vi "Init SPI.vi"(6 "SPI Config":T1={"Mode"=0, "Data Bits"=8, "TX GPIO"=7, "RX GPIO"=4, "SCK GPIO"=6}, 7 "SPI #":T4=-1, 8 "error in (no error)":errorcluster, 10 "Baud":u32=1000000 format="%.0p", 11 "VisaSession in":refnum<class "VisaSession.lvclass">) -> (0 "error out":errorcluster, 2 "SPI":refnum<class "SPI.lvclass">, 3 "VisaSession out":refnum<class "VisaSession.lvclass">)   [LabVIEW 2020, in "CTI.lvlib" / "VisaSession.lvclass"]
uses:
  VisaSession.lvclass
  VisaSession.lvclass/VisaSession.ctl
  Session/Session.lvclass
  SPI Number.ctl
  CTI.lvlib
  GPIO Number.ctl
  SPI Mode.ctl
  SPI Config.ctl
  SPI/SPI.lvclass
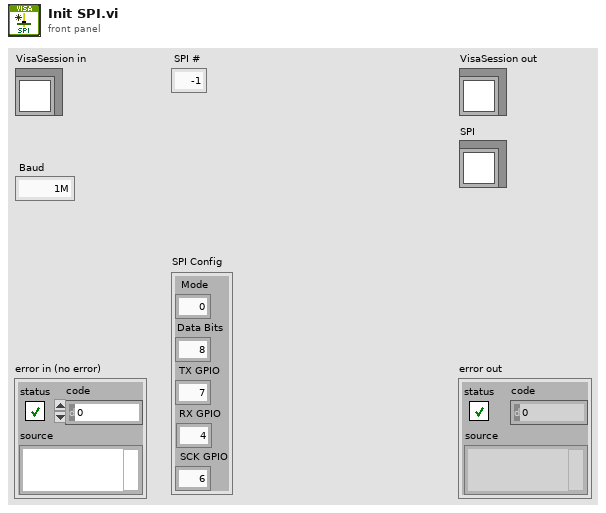
[diagram p1: front panel]
types:
  T1 = typedef "CTI.lvlib/SPI Config.ctl" = cluster{"Mode":T2, "Data Bits":i8, "TX GPIO":T3, "RX GPIO":T3, "SCK GPIO":T3}
  T2 = typedef "CTI.lvlib/SPI Mode.ctl" = i8
  T3 = typedef "CTI.lvlib/GPIO Number.ctl" = i8
  T4 = typedef "CTI.lvlib/SPI Number.ctl" = i8
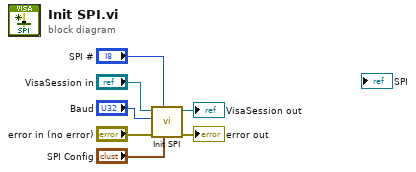
[diagram p0: block diagram]
diagram:
  n1 = call-parent "Init SPI.vi"("SPI Config"="SPI Config", "SPI #"="SPI #", "error in (no error)"="error in (no error)", "Baud"="Baud", "Session in"="VisaSession in") -> ("error out"=→"error out":errorcluster, "Session out"=→"VisaSession out":refnum<class "VisaSession.lvclass">)  [unwired: 4 in, 1 out]
